vi "GenerateFilePath.vi"(8 "Error In":errorcluster, 11 "AutoData":T1) -> (0 "Error Out":errorcluster, 3 "AutoData out":T1)   [LabVIEW 2019, in "AutoMode.lvlib"]
uses:
  AutoMode.lvlib
  Cluster - AutoModeData.ctl
  MainController/Cluster - TestSettings.ctl
  MainController/Cluster - HardwareConfiguration.ctl
  MainController/Cluster - TestResults.ctl
  Cluster - AutoModeMessage.ctl
  Enum - AutoModeState.ctl
  MainController/Cluster - MainControllerMessage.ctl
  MainController/Enum - MainState.ctl
  Utilites/Utilities.lvlib
  MainController/MainController.lvlib
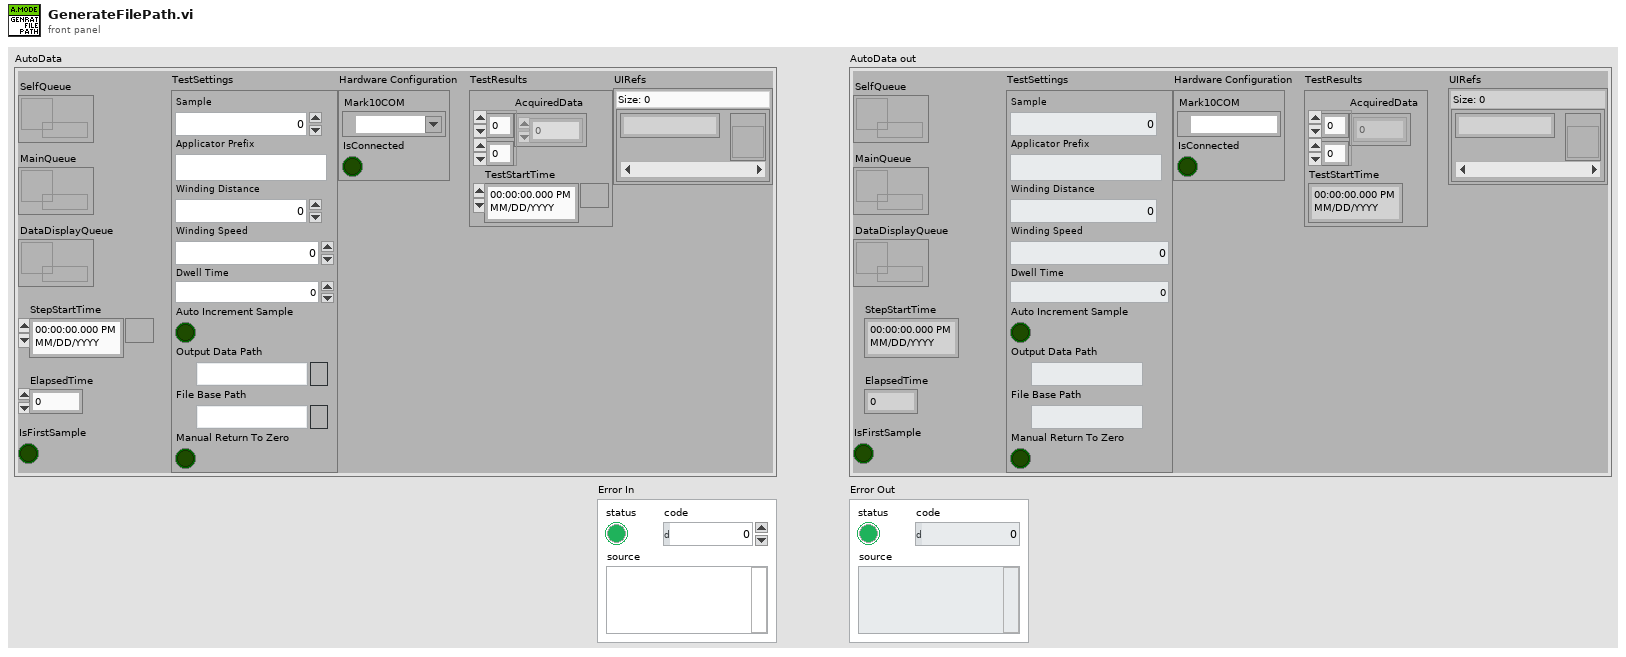
[diagram p1: front panel]
types:
  T1 = typedef "AutoMode.lvlib/Cluster - AutoModeData.ctl" = cluster{"DataDisplayQueue":refnum<queue>, "StepStartTime":timestamp, "TestSettings":T2, "Hardware Configuration":T3, "TestResults":T4, "ElapsedTime":dbl, "IsFirstSample":bool, "UIRefs":map{string, refnum<vi>}, "SelfQueue":refnum<queue>, "MainQueue":refnum<queue>}
  T2 = typedef "MainController.lvlib/Cluster - TestSettings.ctl" = cluster{"Sample":u32, "Applicator Prefix":string, "Winding Distance":dbl, "Winding Speed":dbl, "Dwell Time":dbl, "Auto Increment Sample":bool, "Output Data Path":path, "File Base Path":path, "Manual Return To Zero":bool}
  T3 = typedef "MainController.lvlib/Cluster - HardwareConfiguration.ctl" = cluster{"Mark10COM":refnum<visa-resource-name>, "IsConnected":bool}
  T4 = typedef "MainController.lvlib/Cluster - TestResults.ctl" = cluster{"AcquiredData":dbl[][], "TestStartTime":timestamp}
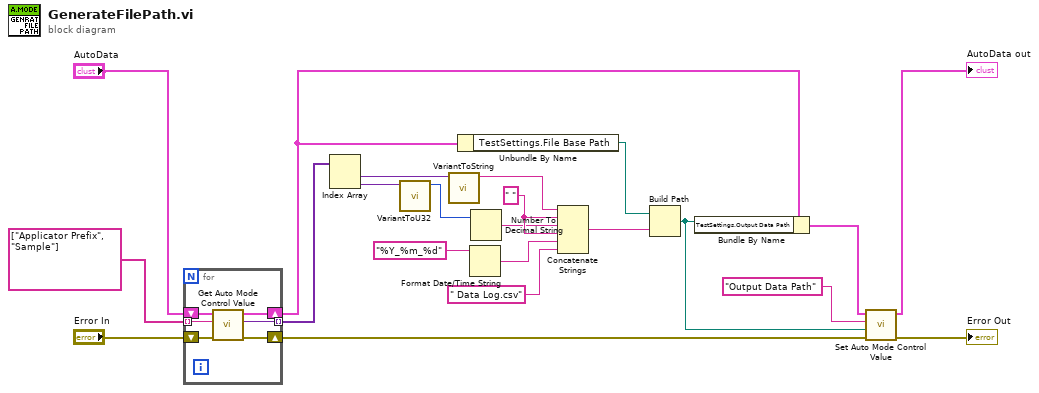
[diagram p0: block diagram]
diagram:
  w21 = " " ("string")
  n1 = for {
    tunnel: string[] ["Applicator Prefix", "Sample"] ("key") -> [w26] mode=indexing
    shift-right: [w27] -> w14
    shift-left: "Error In" -> [w28]
    shift-right: [w24] -> w6
    shift-left: "AutoData" -> [w25]
    tunnel: [w23] -> w11 mode=indexing
    n2 = call "Get Auto Mode Control Value.vi"("Error In"=w28, "key"=w26, "AutoData"=w25) -> ("Error Out"=w27:errorcluster, "Value"=w23:variant, "AutoData out"=w24:T1)  [unwired: 6 in]
  }
  n3 = Index Array(array=w11) -> (element #1=w10:variant, element #2=w8:variant)  [unwired: 2 in]
  n4 = call "VariantToU32.vi"("Variant"=w8) -> ("Value"=w7:u32)  [unwired: 9 in, 1 out]
  n5 = call "VariantToString.vi"("Variant"=w10) -> ("Value"=w9:string)  [unwired: 9 in, 1 out]
  n6 = Unbundle By Name(w6) -> ("TestSettings.File Base Path"=w15:path)
  n7 = Format Date/Time String(time format string (%c)="%Y_%m_%d") -> (date/time string=w20:string)  [unwired: 2 in]
  n8 = Number To Decimal String(number=w7) -> (decimal integer string=w16:string)  [unwired: 1 in]
  n9 = Concatenate Strings(w9, w21, w16, w21, w20, " Data Log.csv" ("string")) -> (w17:string)
  n10 = Build Path(base path=w15, name or relative path=w17) -> (appended path=w1:path)
  n11 = Bundle By Name(cluster=w6, "TestSettings.Output Data Path"=w1) -> (w4:T1)
  n12 = call "Set Auto Mode Control Value.vi"("Error In"=w14, "Value"=w1, "key"="Output Data Path", "AutoData"=w4) -> ("Error Out"=→"Error Out":errorcluster, "AutoData out"=→"AutoData out":T1)  [unwired: 6 in]
